vi "ReceiveTcpMessage.vi"(6 "timeout (5 sec)":i32=5000, 7 "file":bool, 8 "error in (no error)":errorcluster, 11 "connection ID in":T4) -> (0 "error out":errorcluster, 1 "timed out":bool, 2 "message":T1, 3 "connection ID out":T4, 4 "bytes received":i32, 5 "ByteReadErrors":bool[](array[boolean]))   [LabVIEW 2017]
uses:
  <vilib>/addons/InsightCM/MessageBus/TcpApi/controls/TcpMessageReference.ctl
  <vilib>/addons/InsightCM/MessageBus/Base/controls/Message.ctl
  <vilib>/addons/InsightCM/MessageBus/Base/controls/MessageHeader.ctl
  <vilib>/addons/InsightCM/MessageBus/Base/controls/KeyValuePair.ctl
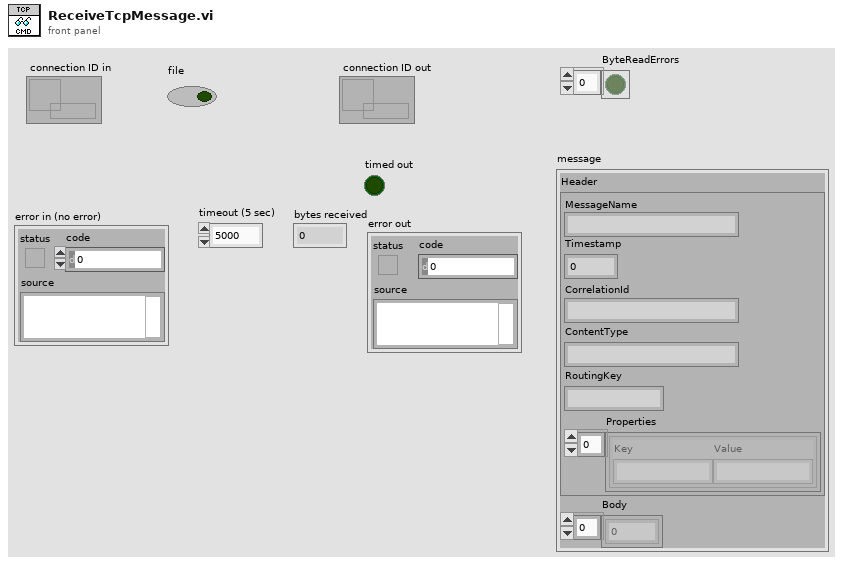
[diagram p1: front panel]
types:
  T1 = typedef "Message.ctl" = cluster{"Header":T2, "Body":u8[]}
  T2 = typedef "MessageHeader.ctl" = cluster{"MessageName":string, "Timestamp":i64, "CorrelationId":string, "ContentType":string, "RoutingKey":string, "Properties":T3[]}
  T3 = typedef "KeyValuePair.ctl" = cluster{"Key":string, "Value":string}
  T4 = typedef "TcpMessageReference.ctl" = refnum<data-value>
  T5 = cluster{"DeviceId":string, "CmdStream":refnum<k5>, "FileStream":refnum<k5>}
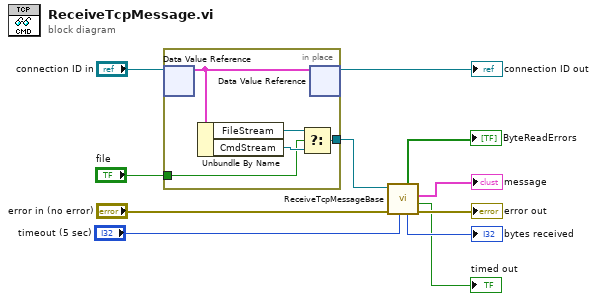
[diagram p0: block diagram]
diagram:
  n1 = in-place {
    in-place-border: "file" -> [w13]
    in-place-border: [w12] -> w8
    n2 = in-place-dvr #1("connection ID in") -> (w16:T5)  [unwired: 1 out]
    n3 = Unbundle By Name(w16) -> ("FileStream"=w15:refnum<k5>, "CmdStream"=w14:refnum<k5>)
    n4 = Select(t=w15, s=w13, f=w14) -> (s? t:f=w12:refnum<k5>)
    n5 = in-place-dvr #1(w16) -> (→"connection ID out":T4)  [unwired: 1 out]
  }
  n6 = call <vilib>:"ReceiveTcpMessageBase.vi"("timeout (5 sec)"="timeout (5 sec)", "error in (no error)"="error in (no error)", "tcp in"=w8) -> ("error out"=→"error out":errorcluster, "timed out"=→"timed out":bool, "Message"=→"message":T1, "bytes received"=→"bytes received":i32, "ByteReadErrors"=→"ByteReadErrors":bool[])  [unwired: 3 in, 1 out]
